vi "Post_Dust_Event_Tick.vi"(7 "error in (no error)":errorcluster, 9 "Small?":bool, 10 "Input Data":T1 {"Estimate Source" items=["Any Source."=-2, "No Shot"=-1, "Basic Labview Estimate"=0, "IDL Estimate From Andrew"=1, "IDL Estimate From Tobin"=2, "Old Metadata"=3]}) -> (0 "error out":errorcluster)   [LabVIEW 2013]
uses:
  Dust_Event.ctl
  Signal.ctl
  Private/Controls/Role ID.ctl
  Private/Controls/Hardware ID.ctl
  Private/Controls/Estimate_source.ctl
panel:
  # "Dust Event"
  # "Signal"
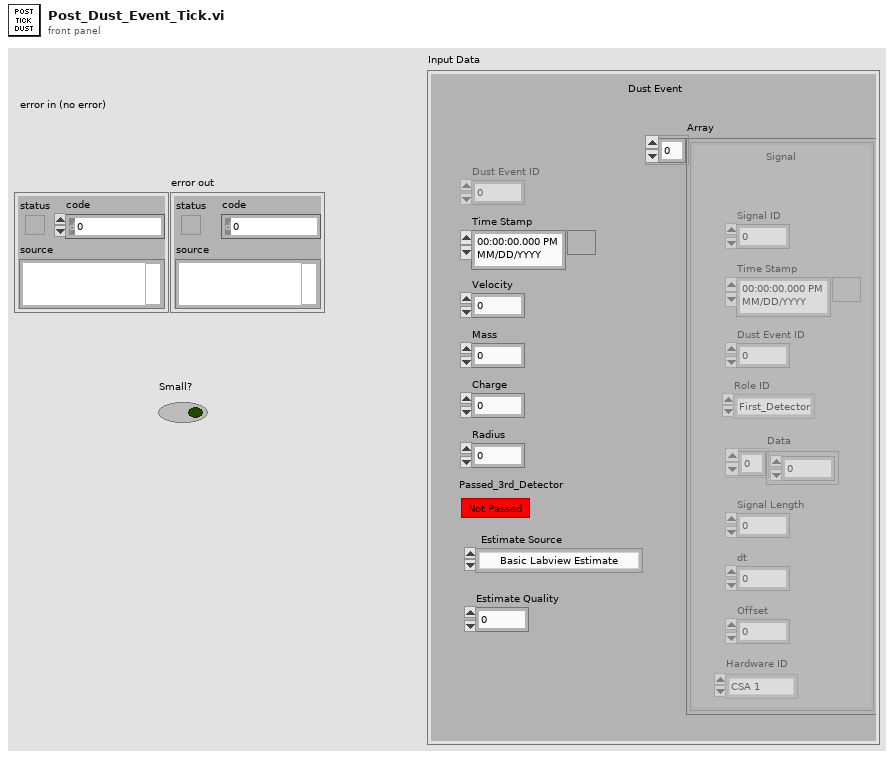
[diagram p1: front panel]
types:
  T1 = typedef "Dust_Event.ctl" = cluster{"Time Stamp":timestamp, "Velocity":sgl, "Mass":sgl, "Charge":sgl, "Radius":sgl, "Array":T2[], "Dust Event ID":i64, "Passed_3rd_Detector":bool, "Estimate Source":T5, "Estimate Quality":sgl}
  T2 = typedef "Signal.ctl" = cluster{"Signal ID":i64, "Time Stamp":timestamp, "Dust Event ID":i64, "Role ID":T3, "Data":sgl[], "Signal Length":i32, "dt":sgl, "Offset":dbl, "Hardware ID":T4}
  T3 = typedef "Role ID.ctl" = enum16{"First_Detector", "Second_Detector", "Third_Detector", "LeCroy_CH1", "LeCroy_CH2", "LeCroy_CH3", "LeCroy_CH4", "PSU"}
  T4 = typedef "Hardware ID.ctl" = enum16{"Unknown", "CSA 1", "CSA 2", "CSA 3", "CSA 4", "CSA 5", "CSA 6"}
  T5 = typedef "Estimate_source.ctl" = i8
  T6 = typedef "Semaphore RefNum" = refnum<k1>
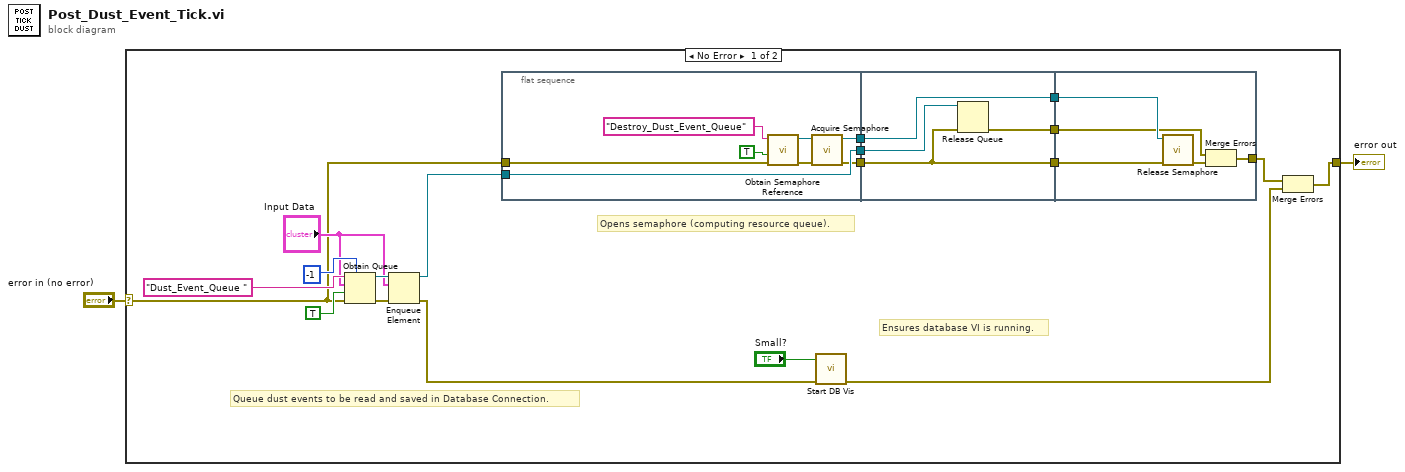
[diagram p0: block diagram]
diagram:
  n1 = case shown="No Error" "error in (no error)" {
    selector: "error in (no error)" -> [w14 w39]
    tunnel: [w6 w39] -> w1
    frame No Error {
      # "Queue dust events to be read and saved in Database Connection."
      # "Opens semaphore (computing resource queue)."
      # "Ensures database VI is running."
      n2 = Obtain Queue(max queue size (-1, unlimited)=-1, name (unnamed)="Dust_Event_Queue ", element data type="Input Data", create if not found? (T)=TRUE, error in (no error)=w14) -> (queue out=w21:refnum<queue>, error out=w15:errorcluster)  [unwired: 1 out]
      n3 = Enqueue Element(queue=w21, element="Input Data", error in (no error)=w15) -> (queue out=w17:refnum<queue>, error out=w5:errorcluster)  [unwired: 1 in, 1 out]
      n4 = flat-sequence {
        tunnel: w14 -> [w24]
        tunnel: w17 -> [w29]
        tunnel: [w29] -> w13
        tunnel: [w23] -> w12
        tunnel: [w22] -> w10
        tunnel: w13 -> [w33]
        tunnel: w12 -> [w30]
        tunnel: [w32] -> w11
        tunnel: w10 -> [w31]
        tunnel: [w31] -> w9
        tunnel: [w30] -> w8
        tunnel: [w34] -> w7
        tunnel: w11 -> [w36]
        tunnel: w9 -> [w37]
        tunnel: w8 -> [w38]
        frame #0 {
          n5 = call <vilib>:"Obtain Semaphore Reference.vi"("error in (no error)"=w24, "create if not found (T)"=TRUE, "name (unnamed)"="Destroy_Dust_Event_Queue") -> ("error out"=w26:errorcluster, "semaphore"=w25:T6)  [unwired: 2 in, 1 out]
          n6 = call <vilib>:"Acquire Semaphore.vi"("error in (no error)"=w26, "semaphore"=w25) -> ("error out"=w23:errorcluster, "semaphore out"=w22:T6)  [unwired: 3 in, 1 out]
        }
        frame #1 {
          n7 = Release Queue(queue=w33, error in (no error)=w30) -> (error out=w32:errorcluster)  [unwired: 1 in, 2 out]
        }
        frame #2 {
          n8 = call <vilib>:"Release Semaphore.vi"("error in (no error)"=w38, "semaphore"=w37) -> ("error out"=w35:errorcluster)  [unwired: 4 in, 1 out]
          n9 = Merge Errors(w36, w35) -> (w34:errorcluster)
        }
      }
      n10 = call "Start DB Vis.vi"("error in (no error)"=w5, "Small?"="Small?") -> ("error out"=w4:errorcluster)  [unwired: 9 in]
      n11 = Merge Errors(w7, w4) -> (w6:errorcluster)
    }
    frame Error {
    }
  }
  "error out" <- w1
